vi "AdaptToInputs.vi"(0 "XRef":T8, 1 "Term Types":T5, 2 "State In":T1) -> (14 "Reply":T3, 15 "Fatal Error Out":T2, 16 "State Out":T1)   [LabVIEW 2017, in "WriteTag.xnode"]
doc: "Write Tag XNode script that adapts the node's terminals to the data types wired to its inputs."
uses:
  WriteTag.xnode
  <vilib>/XNodeSupport/XNodeXNodeRef.ctl
  <vilib>/XNodeSupport/XNodeTermTypeIDPairs.ctl
  <vilib>/XNodeSupport/XNodeTermTypeIDPair.ctl
  <vilib>/XNodeSupport/XNodeType.ctl
  <vilib>/XNodeSupport/XNodeString.ctl
  State.ctl
  <vilib>/XNodeSupport/XNodeStringArray.ctl
  <vilib>/XNodeSupport/XNodeErrorCluster.ctl
  <vilib>/XNodeSupport/NI_XNodeSupport.lvlib
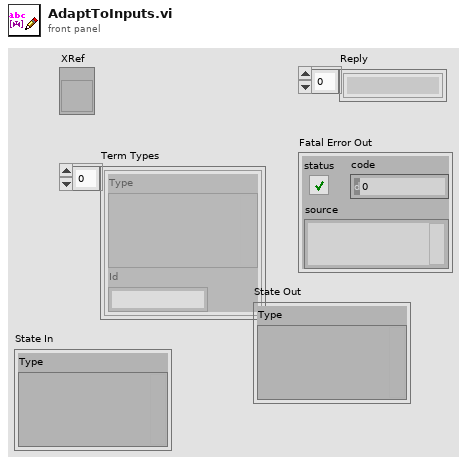
[diagram p1: front panel]
types:
  T1 = typedef "WriteTag.xnode/State.ctl" = cluster{"Type":variant}
  T2 = typedef "NI_XNodeSupport.lvlib/XNodeErrorCluster.ctl" = errorcluster
  T3 = typedef "NI_XNodeSupport.lvlib/XNodeStringArray.ctl" = T4[]
  T4 = typedef "NI_XNodeSupport.lvlib/XNodeString.ctl" = string
  T5 = typedef "NI_XNodeSupport.lvlib/XNodeTermTypeIDPairs.ctl" = T6[]
  T6 = typedef "NI_XNodeSupport.lvlib/XNodeTermTypeIDPair.ctl" = cluster{"Type":T7, "Id":T4}
  T7 = typedef "NI_XNodeSupport.lvlib/XNodeType.ctl" = variant
  T8 = typedef "NI_XNodeSupport.lvlib/XNodeXNodeRef.ctl" = refnum<vi>
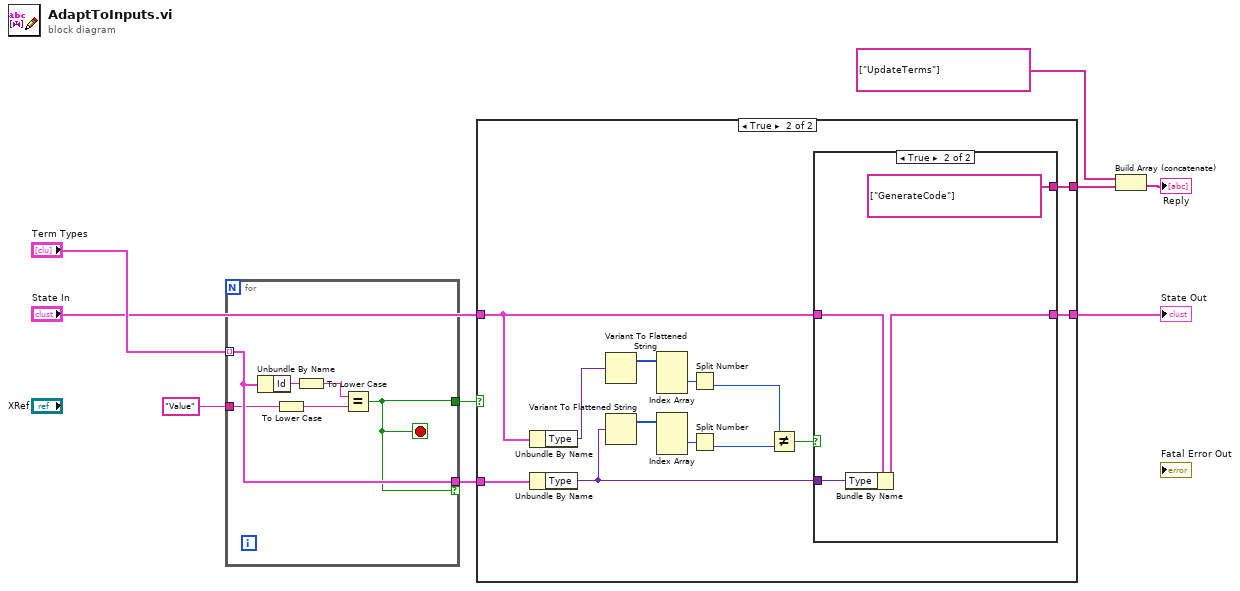
[diagram p0: block diagram]
diagram:
  n1 = for {
    tunnel: "Term Types" -> [w15] mode=indexing
    tunnel: [w15] -> w8 if=w12
    tunnel: "Value" -> [w13]
    tunnel: [w12] -> w7
    stop <- w12 stop-if-true
    n2 = Unbundle By Name(w15) -> ("Id"=w14:T4)
    n3 = To Lower Case(string=w13) -> (all lower case string=w10:string)
    n4 = To Lower Case(string=w14) -> (all lower case string=w11:T4)
    n5 = Equal?(x=w11, y=w10) -> (x = y?=w12:bool)
  }
  n6 = case shown="True" w7 {
    tunnel: [_ w29] -> w3
    tunnel: [w16 w28] -> w4
    tunnel: w8 -> [_ w27]
    tunnel: "State In" -> [w16 w26]
    frame False {
    }
    frame True {
      n7 = Unbundle By Name(w26) -> ("Type"=w20:variant)
      n8 = Unbundle By Name(w27) -> ("Type"=w19:T7)
      n9 = Variant To Flattened String(Variant=w20) -> (1:w24:i16[])  [unwired: 1 out]
      n10 = Variant To Flattened String(Variant=w19) -> (1:w21:i16[])  [unwired: 1 out]
      n11 = Index Array(array=w24) -> (element #2=w23:i16)  [unwired: 3 in, 2 out]
      n12 = Index Array(array=w21) -> (element #2=w22:i16)  [unwired: 3 in, 2 out]
      n13 = Split Number(x=w23) -> (lo(x)=w18:u8)  [unwired: 1 out]
      n14 = Split Number(x=w22) -> (lo(x)=w17:u8)  [unwired: 1 out]
      n15 = Not Equal?(x=w18, y=w17) -> (x != y?=w25:bool)
      n16 = case shown="True" w25 {
        tunnel: [_ T3 ["GenerateCode"] ("Reply")] -> w29
        tunnel: [w30 w33] -> w28
        tunnel: w26 -> [w30 w32]
        tunnel: w19 -> [_ w31]
        frame False {
        }
        frame True {
          n17 = Bundle By Name(cluster=w32, "Type"=w31) -> (w33:T1)
        }
      }
    }
  }
  "State Out" <- w4
  n18 = Build Array (concatenate)(T3 ["UpdateTerms"] ("Reply"), w3) -> (→"Reply":T3)
